vi "Save-log-file.vi"(8 "error in (no error)":errorcluster, 11 "Errors in":T1) -> (0 "error out":errorcluster, 3 "Errors out":T1)   [LabVIEW 2013, in "CameraVision.lvlib" / "CV-Errors.lvclass"]
uses:
  CV-Errors.lvclass
  Object-reference.ctl
  CV-Errors.lvclass/CV-Errors.ctl
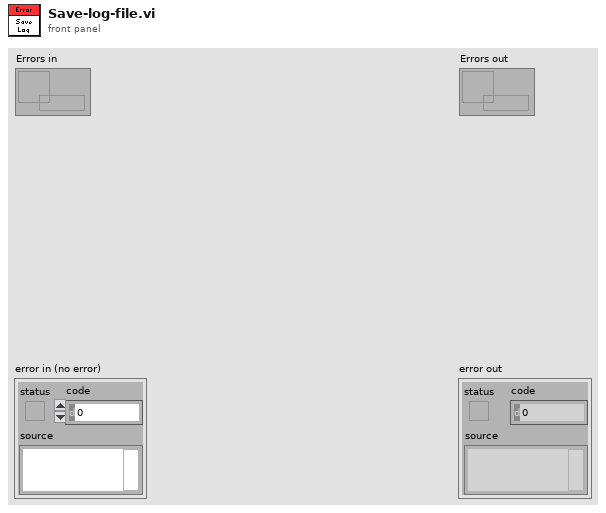
[diagram p1: front panel]
types:
  T1 = typedef "CameraVision.lvlib/CV-Errors.lvclass/Object-reference.ctl" = refnum<data-value>
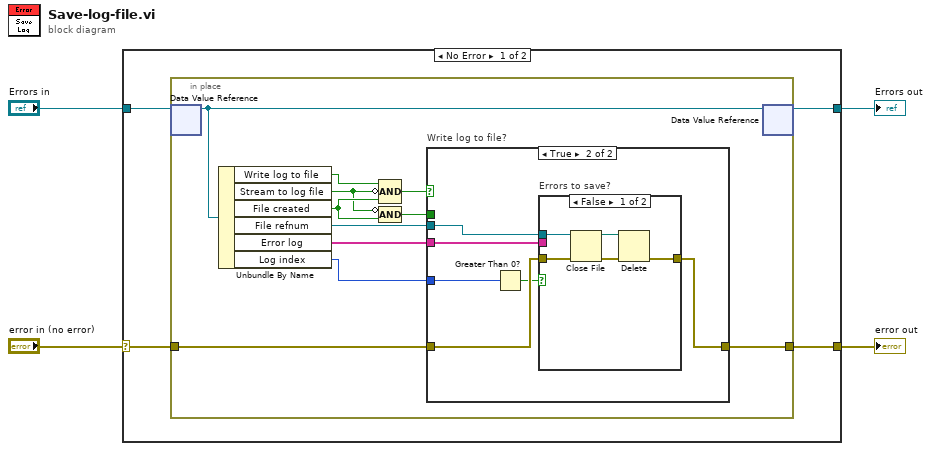
[diagram p0: block diagram]
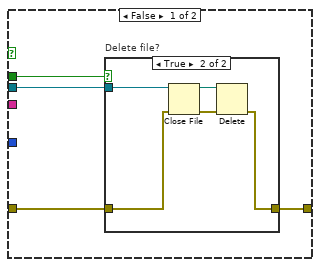
[diagram p2: hidden frame]
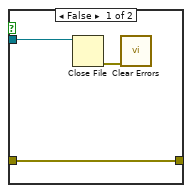
[diagram p3: hidden frame]
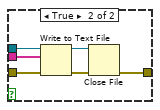
[diagram p4: hidden frame]
diagram:
  n1 = case shown="No Error" "error in (no error)" {
    selector: "error in (no error)" -> [w8 w50]
    tunnel: [w7 w50] -> w3
    tunnel: [w5 w49] -> w1
    tunnel: "Errors in" -> [w6 w49]
    frame No Error {
      n2 = in-place {
        in-place-border: w8 -> [w19]
        in-place-border: [w13] -> w7
        n3 = in-place-dvr #1(w6) -> (w11:refnum<class "CV-Errors.lvclass">)  [unwired: 1 out]
        n4 = Unbundle By Name(w11) -> ("Write log to file"=w15:bool, "Stream to log file"=w9:bool, "File created"=w14:bool, "File refnum"=w16:refnum<file>, "Error log"=w17:string[], "Log index"=w12:i32)
        n5 = Compound Arithmetic op=AND(w15, invert w9, w14) -> (w18:bool)
        n6 = Compound Arithmetic op=AND(invert w9, w14) -> (w10:bool)
        n7 = case "Write log to file?" shown="True" w18 {
          tunnel: w19 -> [w22 w37]
          tunnel: [w21 w35] -> w13
          tunnel: w16 -> [w23 w36]
          tunnel: w17 -> [_ w34]
          tunnel: w10 -> [w20 _]
          tunnel: w12 -> [_ w32]
          frame False {
            n8 = case "Delete file?" shown="True" w20 {
              tunnel: w23 -> [w25 w31]
              tunnel: w22 -> [w26 w30]
              tunnel: [w26 w28] -> w21
              frame False {
                n9 = Close File(refnum=w25) -> (error out=w24:errorcluster)  [unwired: 1 in, 1 out]
                n10 = call <vilib>:"Clear Errors.vi"("error in (no error)"=w24) -> ()  [unwired: 6 in, 1 out]
              }
              frame True {
                n11 = Close File(refnum=w31, error in=w30) -> (path=w27:path, error out=w29:errorcluster)
                n12 = Delete(path (use dialog)=w27, error in=w29) -> (error out=w28:errorcluster)  [unwired: 3 in, 2 out]
              }
            }
          }
          frame True {
            n13 = Greater Than 0?(x=w32) -> (x > 0?=w33:bool)
            n14 = case "Errors to save?" shown="False" w33 {
              tunnel: w37 -> [w42 w48]
              tunnel: w36 -> [w41 w47]
              tunnel: w34 -> [_ w46]
              tunnel: [w39 w43] -> w35
              frame False {
                n15 = Close File(refnum=w41, error in=w42) -> (path=w38:path, error out=w40:errorcluster)
                n16 = Delete(path (use dialog)=w38, error in=w40) -> (error out=w39:errorcluster)  [unwired: 3 in, 2 out]
              }
              frame True {
                n17 = Write to Text File(file (use dialog)=w47, text=w46, error in=w48) -> (refnum out=w45:refnum<file>, error out=w44:errorcluster)  [unwired: 1 in, 1 out]
                n18 = Close File(refnum=w45, error in=w44) -> (error out=w43:errorcluster)  [unwired: 1 out]
              }
            }
          }
        }
        n19 = in-place-dvr #1(w11) -> (w5:T1)  [unwired: 1 out]
      }
    }
    frame Error {
    }
  }
  "error out" <- w3
  "Errors out" <- w1
